vi "Calculate GRR Core.vi"(8 "error in (no error)":errorcluster, 11 "Test Data":T2[](array[typedef])) -> (0 "error out":errorcluster, 3 "Result Data":T1[](array[typedef]))   [LabVIEW 2018, in "GRR Core.lvclass"]
uses:
  GRR Core.lvclass
  TestDataMgr/Typedefs/Test Data All.ctl
  TestDataMgr/Typedefs/Test Limits.ctl
  TestDataMgr/Typedefs/Test Raw Data.ctl
  Result Data Mgr/Typedefs/GRR Result.ctl
  Typedefs/Calculation Info.ctl
  <vilib>/Analysis/baseanly.llb/Mean (DBL).vi
  <vilib>/Analysis/NI_AALBase.lvlib
  Result Data Mgr/Result Data Mgr.lvclass
  TestDataMgr/TestDataMgr.lvclass
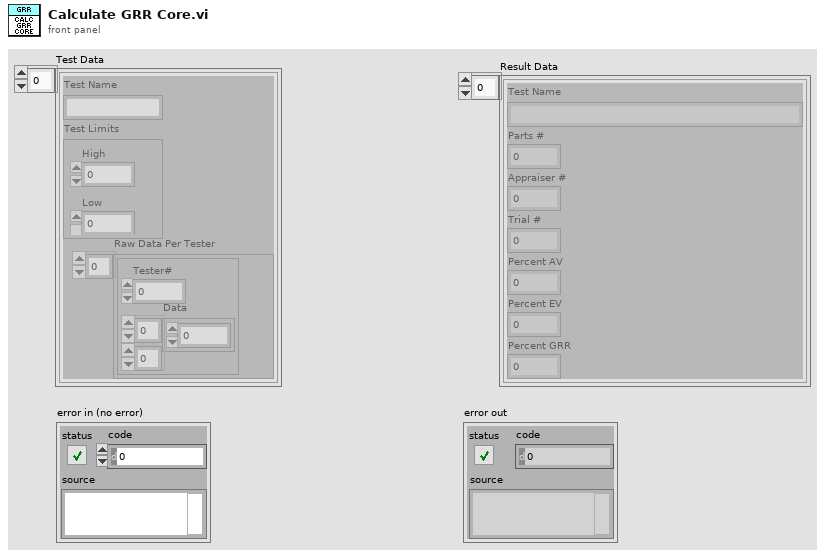
[diagram p1: front panel]
types:
  T1 = typedef "Result Data Mgr.lvclass/GRR Result.ctl" = cluster{"Test Name":string, "Parts #":u8, "Appraiser #":u8, "Trial #":u8, "Percent AV":dbl, "Percent EV":dbl, "Percent GRR":dbl}
  T2 = typedef "TestDataMgr.lvclass/Test Data All.ctl" = cluster{"Test Name":string, "Test Limits":T3, "Raw Data Per Tester":T4[]}
  T3 = typedef "TestDataMgr.lvclass/Test Limits.ctl" = cluster{"High":dbl, "Low":dbl}
  T4 = typedef "TestDataMgr.lvclass/Test Raw Data.ctl" = cluster{"Data":dbl[][], "Tester#":u8}
  T5 = typedef "GRR Core.lvclass/Calculation Info.ctl" = cluster{"Parts #":u8, "Appraisers #":u8, "Trial #":u8}
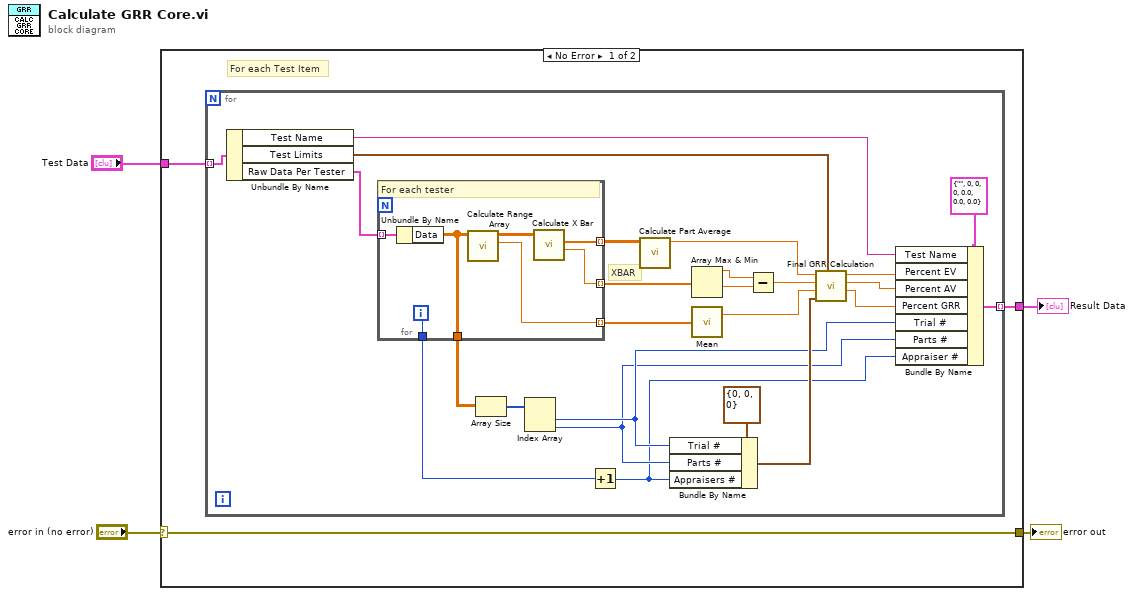
[diagram p0: block diagram]
diagram:
  n1 = case shown="No Error" "error in (no error)" {
    selector: "error in (no error)" -> [w5 w40]
    tunnel: "Test Data" -> [w7 _]
    tunnel: [w6 _] -> w4
    tunnel: [w5 w40] -> w2
    frame No Error {
      # "For each Test Item"
      n2 = for {
        tunnel: w7 -> [w32] mode=indexing
        tunnel: [w8] -> w6 mode=indexing
        # "XBAR"
        n3 = Unbundle By Name(w32) -> ("Test Name"=w15:string, "Test Limits"=w25:T3, "Raw Data Per Tester"=w31:T4[])
        n4 = for {
          tunnel: w31 -> [w39] mode=indexing
          tunnel: [w37] -> w26 mode=indexing
          tunnel: [w36] -> w30 mode=indexing
          tunnel: [w35] -> w27 mode=indexing
          tunnel: [w34] -> w21
          tunnel: [w33] -> w20
          i -> [w34]
          # "For each tester"
          n5 = Unbundle By Name(w39) -> ("Data"=w33:dbl[][])
          n6 = call "Calculate Range Array.vi"("2D Array In"=w33) -> ("Average Range"=w37:dbl, "2D array Out"=w38:dbl[][])  [unwired: 8 in, 1 out]
          n7 = call "Calculate X Bar.vi"("2D Array In"=w38) -> ("Xbar"=w35:dbl, "Average Array"=w36:dbl[])  [unwired: 8 in, 1 out]
        }
        n8 = Array Size(array=w20) -> (size(s)=w19:i32[])
        n9 = Index Array(array=w19) -> (element #1=w11:i32, element #2=w10:i32)  [unwired: 2 in]
        n10 = Increment(x=w21) -> (x+1=w9:i32)
        n11 = call "Calculate Part Average.vi"("Avg Array"=w30) -> ("Parts Averages"=w24:dbl)  [unwired: 10 in]
        n12 = Bundle By Name(cluster=T5 {"Parts #"=0, "Appraisers #"=0, "Trial #"=0} ("Calc Info"), "Trial #"=w11, "Parts #"=w10, "Appraisers #"=w9) -> (w17:T5)
        n13 = Array Max & Min(array=w27) -> (max value=w29:dbl, min value=w28:dbl)  [unwired: 2 out]
        n14 = call-poly <vilib>:"Mean.vi"("X"=w26) -> ("mean"=w22:dbl)  [unwired: 1 out]
        n15 = Subtract(x=w29, y=w28) -> (x-y=w23:dbl)
        n16 = call "Final GRR Calculation.vi"("Test Limits"=w25, "Calc Info"=w17, "R Double Bar"=w22, "X Bar Diff"=w23, "Rp"=w24) -> ("Percent GRR"=w12:dbl, "Percent AV"=w13:dbl, "Percent EV"=w14:dbl)  [unwired: 4 in]
        n17 = Bundle By Name(cluster=T1 {"Test Name"="", "Parts #"=0, "Appraiser #"=0, "Trial #"=0, "Percent AV"=0.0, "Percent EV"=0.0, "Percent GRR"=0.0} ("GRR Results"), "Test Name"=w15, "Percent EV"=w14, "Percent AV"=w13, "Percent GRR"=w12, "Trial #"=w11, "Parts #"=w10, "Appraiser #"=w9) -> (w8:T1)
      }
    }
    frame Error {
    }
  }
  "Result Data" <- w4
  "error out" <- w2
